vi "Routes.vi"(7 "Action":T1, 9 "Navbar Page? (F)":bool, 10 "Endpoint in":string, 11 "Path":string) -> (1 "Is Navbar Page?":bool, 2 "Endpoint out":string, 3 "Found?":bool, 5 "Paths":string[](array[string]))   [LabVIEW 2021, in "HttpServer.lvlib"]
uses:
  HttpServer.lvlib
  TypeDefs/Action.ctl
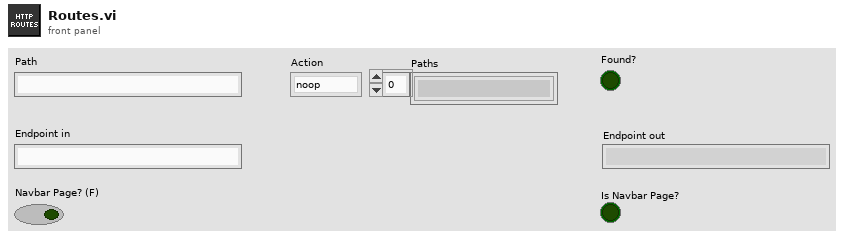
[diagram p1: front panel]
types:
  T1 = typedef "HttpServer.lvlib/Action.ctl" = enum8{"noop", "add", "get", "set", "remove"}
  T2 = map{string, cluster{"Endpoint":string, "IsPage":bool}}
  T3 = cluster{"Endpoint in":string, "Navbar Page? (F)":bool}
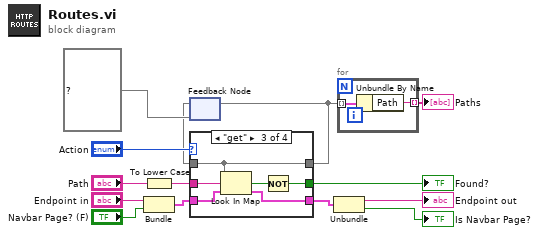
[diagram p0: block diagram]
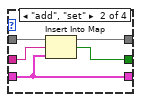
[diagram p3: hidden frame]
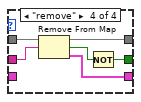
[diagram p4: hidden frame]
diagram:
  n1 = To Lower Case(string="Path") -> (all lower case string=w5:string)
  n2 = Bundle("Endpoint in"="Endpoint in", "Navbar Page? (F)"="Navbar Page? (F)") -> (w4:T3)  [unwired: 1 in]
  n3 = feedback #1(T2 {} ("Routes")) -> (w12:T2)
  n4 = case shown="\"get\"" "Action" {
    tunnel: w12 -> [w15 w20 w26 w32]
    tunnel: [w15 w19 w26 w31] -> w10
    tunnel: w5 -> [_ w18 w25 w30]
    tunnel: w4 -> [_ w16 w24 _]
    tunnel: [_ w16 w23 w29] -> w6
    tunnel: [_ w17 w21 w27] -> w8
    frame "noop" {
    }
    frame "add", "set" {
      n5 = Insert Into Map(map in=w20, key=w18, value=w16) -> (map out=w19:T2, key already included?=w17:bool)  [unwired: 1 out]
    }
    frame "get" {
      n6 = Look In Map(map=w26, key=w25, default value=w24) -> (key not found?=w22:bool, value=w23:cluster{"Endpoint":string, "IsPage":bool})
      n7 = Not(x=w22) -> (.not. x?=w21:bool)
    }
    frame "remove" {
      n8 = Remove From Map(10:w30, 11:w32) -> (1:w29:cluster{"Endpoint":string, "IsPage":bool}, 2:w28:bool, 3:w31:T2)
      n9 = Not(x=w28) -> (.not. x?=w27:bool)
    }
  }
  "Found?" <- w8
  n10 = feedback-in #1(w10) -> ()
  n11 = Unbundle(w6) -> ("Endpoint"=→"Endpoint out":string, "IsPage"=→"Is Navbar Page?":bool)
  n12 = for {
    tunnel: w10 -> [w34] mode=indexing
    tunnel: [w33] -> w9 mode=indexing
    n13 = Unbundle By Name(w34) -> ("Path"=w33:string)
  }
  "Paths" <- w9
